vi "XYZMovingPartModifying_WangYunong.vi"() -> ()   [LabVIEW 2013]
uses:
  <vilib>/Math Plots/3D Math Plots/3D Bar/3D Bar XCtrl/3D Bar.xctl
  <vilib>/Math Plots/3D Math Plots/3D Bar/3D Bar Datatype/Public/Plot Helper (Matrix).vi
  <vilib>/Instr/_visa.llb/VISA Configure Serial Port (Instr).vi
  <vilib>/Math Plots/3D Math Plots/3D Bar/3D Bar Datatype/3D Bar Datatype.lvclass
panel:
  out "Zvel (mm/s)":dbl
  in  "stop":bool
  in  "Path":path
  out "Current ratio":dbl(graph)
  out "Surface Scanned":refnum<class "3D Plot Datatype.lvclass">[](xcontrol)
  in  "Z step / s":dbl format="%#_13g"
  out "Height / mm":dbl format="%#_13g"
  out "Present I Percent":dbl format="%#_13g"
  out "Present I / A":dbl format="%#_13g"
  in  "mm / step":dbl
  in  "ErrorTolerant %":dbl format="%#_13g"
  out "Reference A":dbl
  in  "VoltageGenerator":refnum<visa-resource-name>
  in  "ZMovingControl":refnum<visa-resource-name>
  out "Rod Pos?":cluster{dbl[], dbl[]}(graph)
  in  "X pole":refnum<visa-resource-name>
  in  "Y pole":refnum<visa-resource-name>
  in  "XYMov speed(mm/s)":dbl format="%#_13g"
  out "y resolution":dbl
  out "x resolution":dbl
  out "XY Graph":cluster{dbl[], dbl[]}(graph)
  in  "Y Center / mm":dbl format="%#_13g"
  in  "X Center / mm":dbl format="%#_13g"
  in  "Size input solution":enum16{"Dynamic Size", "Fixed Size"}(ring)=enum."Fixed Size"
  in  "Shape":enum16{"Self-defined", "Circle"}(ring)=enum."Circle"
  in  "Radius / mm":dbl format="%#_13g"
  in  "Precision":i32
  in  "Polygon Point":dbl[][](array[numeric])
  out "X":i32
  out "Y":i32
  in  "Y move Maximum / mm":dbl
  in  "X move Maximum / mm":dbl
  in  "Y step / mm":dbl
  in  "X step / mm":dbl
  in  "Initial YPos / mm":dbl
  in  "Initial XPos / mm":dbl
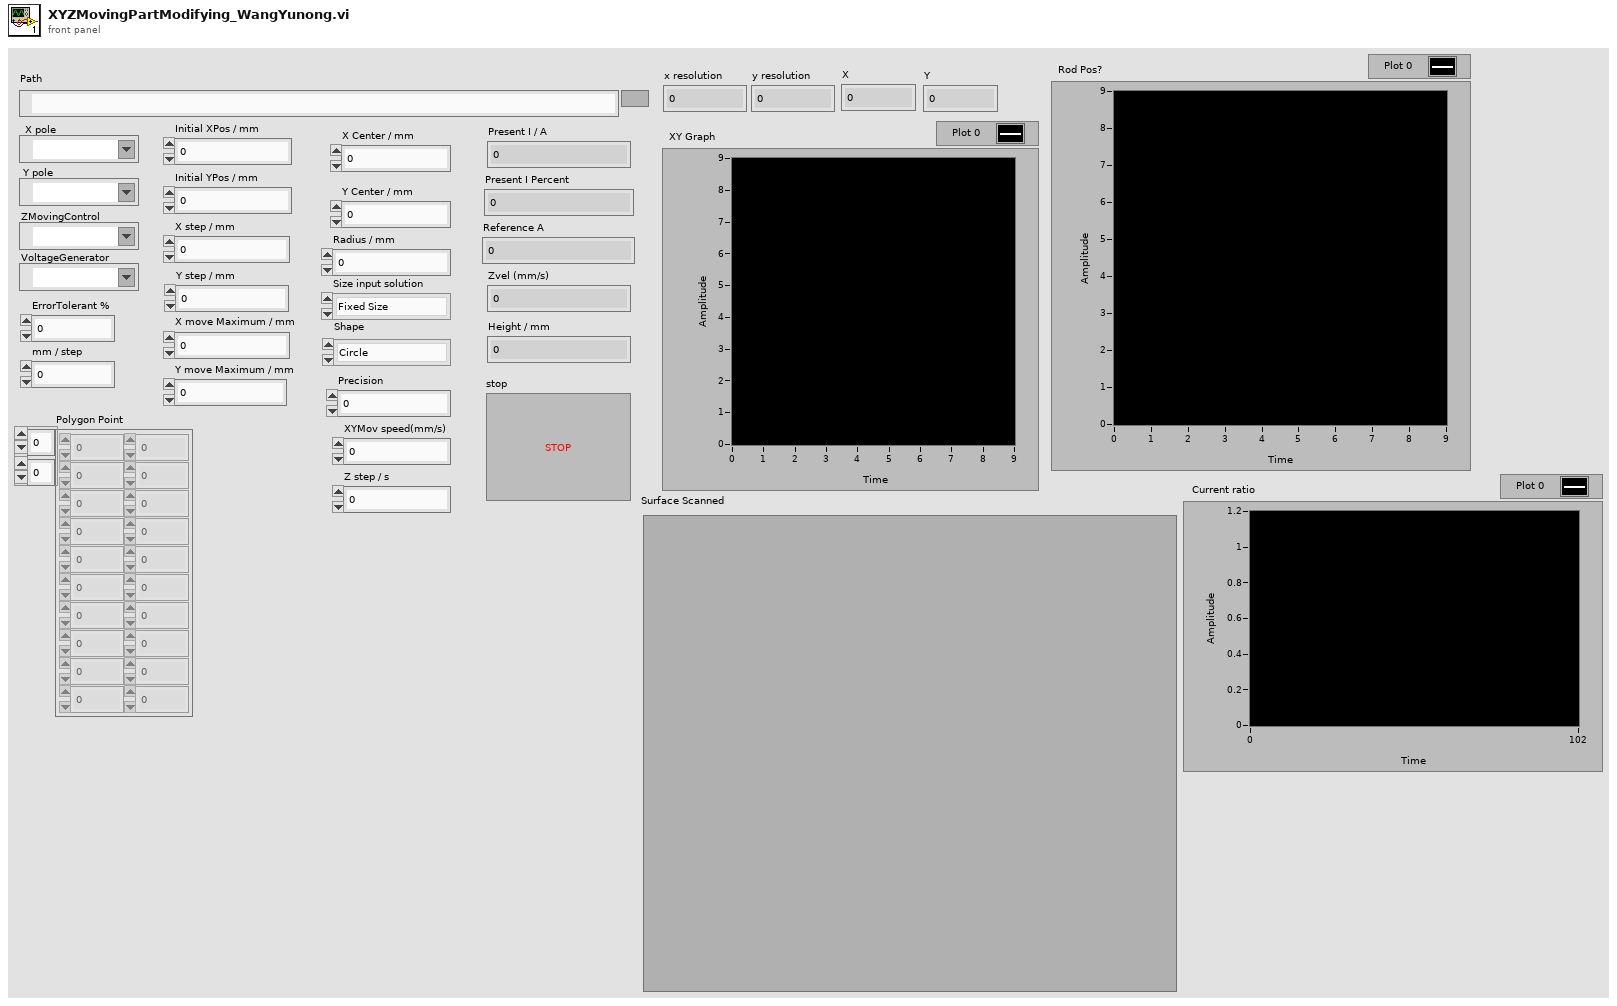
[diagram p1: front panel]
types:
  T1 = enum16{"open", "replace", "create", "open or create", "replace or create", "replace or create with confirmation"}
  T2 = typedef "NI_Matrix.lvlib/RealMatrix.ctl" = dbl[][]
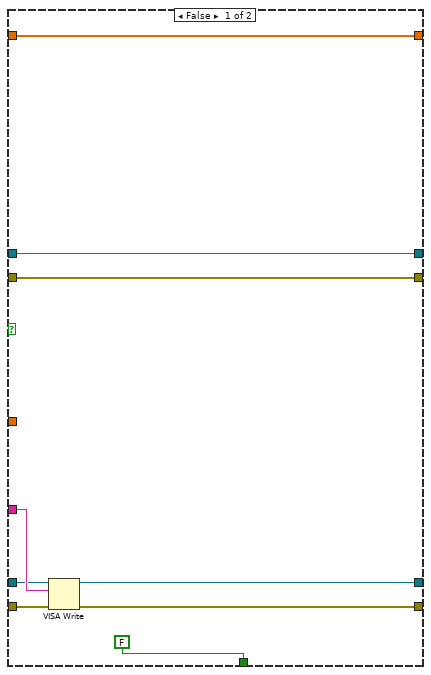
[diagram p3: hidden frame]
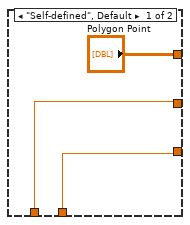
[diagram p4: hidden frame]
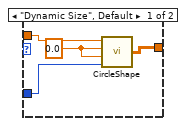
[diagram p5: hidden frame]
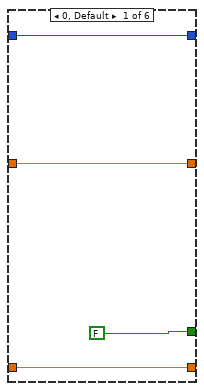
[diagram p6: hidden frame]
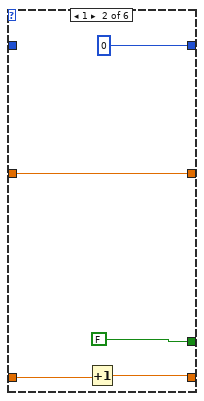
[diagram p7: hidden frame]
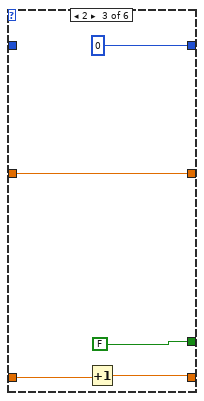
[diagram p8: hidden frame]
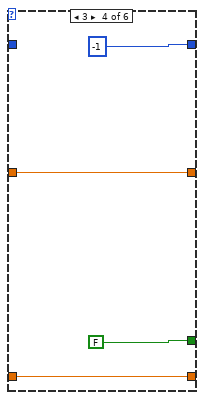
[diagram p9: hidden frame]
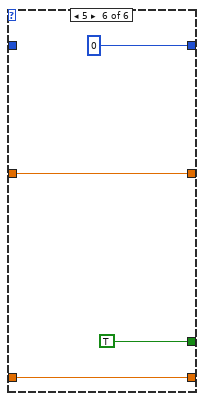
[diagram p10: hidden frame]
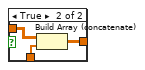
[diagram p11: hidden frame]
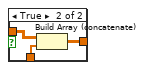
[diagram p12: hidden frame]
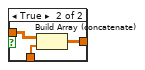
[diagram p13: hidden frame]
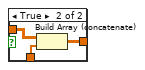
[diagram p14: hidden frame]
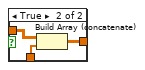
[diagram p15: hidden frame]
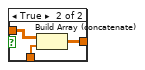
[diagram p16: hidden frame]
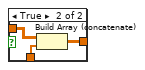
[diagram p17: hidden frame]
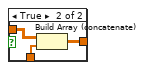
[diagram p18: hidden frame]
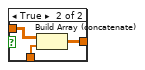
[diagram p19: hidden frame]
diagram:
  w59 = "ERR?\nMOV 1 0\n"
  w30 = dbl[] []
  w125 = 0 ("index")
  w94 = dbl[][] []
  w168 = 0
  w169 = 9.5
  w174 = 5.0
  # "sorted Y pos"
  # "sorted X pos"
  # "Control smallest step of 50nm"
  # "y length"
  # "x length"
  n1 = Greater?(x="Initial XPos / mm", y=w174) -> (0:w173:bool)
  n2 = Greater?(x="Initial YPos / mm", y=w174) -> (0:w172:bool)
  n3 = Or(x=w173, y=w172) -> (x .or. y?=w132:bool)
  n4 = case shown="True" w132 {
    tunnel: "Initial XPos / mm" -> [w176 _]
    tunnel: "Initial YPos / mm" -> [w175 _]
    tunnel: [w176 w177] -> w113
    tunnel: [w175 w177] -> w112
    frame False {
    }
    frame True {
      w177 = 5.0
    }
  }
  n5 = Greater Or Equal?(x=w112, y="Y move Maximum / mm") -> (x >= y?=w156:bool)
  n6 = Greater Or Equal?(x=w113, y="X move Maximum / mm") -> (x >= y?=w157:bool)
  n7 = Or(x=w157, y=w156) -> (x .or. y?=w131:bool)
  n8 = Less Or Equal?(x="Y step / mm", y=w168) -> (x <= y?=w165:bool)
  n9 = Greater Or Equal?(x="Y step / mm", y="Y move Maximum / mm") -> (x >= y?=w164:bool)
  n10 = Greater Or Equal?(x="X step / mm", y="X move Maximum / mm") -> (x >= y?=w166:bool)
  n11 = Less Or Equal?(x="X step / mm", y=w168) -> (x <= y?=w167:bool)
  n12 = Greater?(x="X move Maximum / mm", y=w169) -> (0:w155:bool)
  n13 = Greater?(x="Y move Maximum / mm", y=w169) -> (0:w154:bool)
  n14 = Compound Arithmetic op=OR(w167, w166, w165, w164) -> (w130:bool)
  n15 = case shown="True" w130 {
    tunnel: "X step / mm" -> [w179 _]
    tunnel: "Y step / mm" -> [w178 _]
    tunnel: [w179 w180] -> w153
    tunnel: [w178 w180] -> w152
    frame False {
    }
    frame True {
      w180 = 0.0
    }
  }
  n16 = case shown="True" w155 {
    tunnel: w169 -> [_ w182]
    tunnel: "X move Maximum / mm" -> [w181 _]
    tunnel: [w181 w182] -> w144
    frame False {
    }
    frame True {
    }
  }
  n17 = case shown="True" w154 {
    tunnel: w169 -> [_ w184]
    tunnel: "Y move Maximum / mm" -> [w183 _]
    tunnel: [w183 w184] -> w143
    frame False {
    }
    frame True {
    }
  }
  n18 = call "Intolerable Error 3"("Enable"=w130) -> ()  [unwired: 9 in, 2 out]
  n19 = call "Intolerable Error"("Enable"=w132) -> ()  [unwired: 9 in, 2 out]
  n20 = Subtract(x=w144, y=w113) -> (x-y=w138:dbl)
  n21 = Subtract(x=w143, y=w112) -> (x-y=w137:dbl)
  n22 = case shown="\"Circle\"" "Shape" {
    tunnel: ["Polygon Point" w200] -> w146
    tunnel: "Size input solution" -> [_ w199]
    tunnel: w138 -> [_ w195]
    tunnel: w137 -> [_ w194]
    tunnel: w112 -> [w185 w193]
    tunnel: w113 -> [w186 w192]
    tunnel: [w186 w191] -> w136
    tunnel: [w185 w190] -> w135
    tunnel: "X Center / mm" -> [_ w189]
    tunnel: "Y Center / mm" -> [_ w188]
    frame "Self-defined", Default {
    }
    frame "Circle" {
      w198 = 2.0
      n23 = Divide(x=w194, y=w198) -> (x/y=w196:dbl)
      n24 = Divide(x=w195, y=w198) -> (x/y=w197:dbl)
      n25 = case shown="\"Fixed Size\"" w199 {
        tunnel: "Radius / mm" -> [w205 w211]
        tunnel: "Precision" -> [w204 w210]
        tunnel: [w206 w209] -> w200
        tunnel: w189 -> [_ w208]
        tunnel: w188 -> [_ w207]
        frame "Dynamic Size", Default {
          w203 = 0.0 ("X initial")
          n26 = call "CircleShape.vi"("Precision"=w204, "Y initial"=w203, "X initial"=w203, "Radius"=w205) -> ("Output Point"=w206:dbl[][])
        }
        frame "Fixed Size" {
          n27 = call "CircleShape.vi"("Precision"=w210, "Y initial"=w207, "X initial"=w208, "Radius"=w211) -> ("Output Point"=w209:dbl[][])
        }
      }
      n28 = Add(x=w197, y=w192) -> (x+y=w191:dbl)
      n29 = Add(x=w196, y=w193) -> (x+y=w190:dbl)
    }
  }
  n30 = Index Array(array=w146, index (col)=1 ("disabled index (col)")) -> (element=w115:dbl[])  [unwired: 1 in]
  n31 = Index Array(array=w146, index (col)=0 ("disabled index (col)")) -> (element=w116:dbl[])  [unwired: 1 in]
  n32 = Array Size(array=w116) -> (size(s)=w118:i32)
  n33 = Array Size(array=w115) -> (size(s)=w117:i32)
  n34 = flat-sequence {
    tunnel: w153 -> [w225]
    tunnel: w152 -> [w222]
    tunnel: [w218] -> w54
    tunnel: [w217] -> w53
    frame #0 {
      w214 = 50
      w219 = 1000000.0
      n35 = Multiply(x=w219, y=w222) -> (x*y=w221:dbl)
      n36 = Multiply(x=w225, y=w219) -> (x*y=w224:dbl)
      n37 = Divide(x=w221, y=w214) -> (x/y=w220:dbl)
      n38 = Divide(x=w224, y=w214) -> (x/y=w223:dbl)
      n39 = Round To Nearest(number=w220) -> (nearest integer value=w215:dbl)
      n40 = Round To Nearest(number=w223) -> (nearest integer value=w216:dbl)
      n41 = Multiply(x=w215, y=w214) -> (x*y=w213:dbl)
      n42 = Multiply(x=w216, y=w214) -> (x*y=w212:dbl)
      n43 = Divide(x=w213, y=w219) -> (x/y=w217:dbl)
      n44 = Divide(x=w212, y=w219) -> (x/y=w218:dbl)
    }
  }
  n45 = call "Intolerable Error 4"("Enable"=w129) -> ()  [unwired: 9 in, 2 out]
  n46 = call "Intolerable Error 2"("Enable"=w131) -> ()  [unwired: 9 in, 2 out]
  n47 = call "Tolerable Error"("Enable"=w155) -> ()  [unwired: 9 in, 2 out]
  n48 = Sort 1D Array(array=w116) -> (sorted array=w123:dbl[])
  n49 = Sort 1D Array(array=w115) -> (sorted array=w124:dbl[])
  n50 = Decrement(x=w117) -> (x-1=w126:i32)
  n51 = Decrement(x=w118) -> (x-1=w127:i32)
  n52 = call "Tolerable Error 2"("Enable"=w154) -> ()  [unwired: 9 in, 2 out]
  n53 = Index Array(array=w123, index=w125) -> (element=w122:dbl)
  n54 = Index Array(array=w123, index=w127) -> (element=w121:dbl)
  n55 = Index Array(array=w124, index=w126) -> (element=w120:dbl)
  n56 = Index Array(array=w124, index=w125) -> (element=w119:dbl)
  n57 = flat-sequence {
    tunnel: w138 -> [w248]
    tunnel: w137 -> [w247]
    tunnel: w144 -> [w254]
    tunnel: w113 -> [w231]
    tunnel: w143 -> [w253]
    tunnel: w112 -> [w227]
    tunnel: [w252] -> w129
    tunnel: w54 -> [w230]
    tunnel: w53 -> [w226]
    tunnel: [w251] -> w3
    tunnel: [w229] -> w151
    tunnel: [w228] -> w150
    tunnel: [w226] -> w149
    tunnel: [w230] -> w148
    tunnel: [w246] -> w145
    tunnel: w136 -> [w245]
    tunnel: w135 -> [w244]
    tunnel: w144 -> [w243]
    tunnel: w143 -> [w242]
    tunnel: [w241] -> w140
    tunnel: [w240] -> w141
    tunnel: "Size input solution" -> [w239]
    tunnel: w122 -> [w238]
    tunnel: w121 -> [w237]
    tunnel: w120 -> [w236]
    tunnel: w119 -> [w235]
    tunnel: w116 -> [w234]
    tunnel: w115 -> [w233]
    tunnel: "Shape" -> [w232]
    tunnel: [w231] -> w103
    tunnel: [w230] -> w102
    tunnel: [w229] -> w101
    tunnel: [w228] -> w98
    tunnel: [w227] -> w97
    tunnel: [w226] -> w96
    frame #0 {
      n58 = case shown="\"Dynamic Size\", Default" w239 {
        tunnel: w234 -> [w277 w305]
        tunnel: w233 -> [w276 w304]
        tunnel: w237 -> [w283 w320]
        tunnel: w238 -> [w262 w318]
        tunnel: w236 -> [w282 w316]
        tunnel: w235 -> [w260 w313]
        tunnel: w248 -> [w281 _]
        tunnel: w247 -> [w278 _]
        tunnel: [w263 w306] -> w251
        tunnel: w254 -> [_ w319]
        tunnel: w231 -> [w271 w317]
        tunnel: w253 -> [_ w315]
        tunnel: w227 -> [w270 w314]
        tunnel: [FALSE w307] -> w252
        tunnel: w245 -> [w255 _]
        tunnel: w244 -> [w256 _]
        tunnel: w230 -> [w269 _]
        tunnel: w226 -> [w268 _]
        tunnel: [w266 w303] -> w241
        tunnel: [w267 w303] -> w240
        tunnel: w232 -> [w272 _]
        frame "Dynamic Size", Default {
          n59 = case shown="\"Self-defined\", Default" w272 {
            tunnel: w271 -> [_ w300]
            tunnel: w270 -> [_ w299]
            tunnel: w269 -> [_ w298]
            tunnel: w268 -> [_ w297]
            tunnel: [w289 w296] -> w267
            tunnel: [w289 w295] -> w266
            tunnel: w262 -> [w288 w294]
            tunnel: [w285 w293] -> w261
            tunnel: w260 -> [w287 w292]
            tunnel: [w284 w290] -> w259
            frame "Self-defined", Default {
              w286 = 0
              w289 = 0
              n60 = Multiply(x=w288, y=w286) -> (x*y=w285:dbl)
              n61 = Multiply(x=w286, y=w287) -> (x*y=w284:dbl)
            }
            frame "Circle" {
              w291 = 1.0
              n62 = Divide(x=w299, y=w297) -> (x/y=w301:dbl)
              n63 = Divide(x=w300, y=w298) -> (x/y=w302:dbl)
              n64 = Multiply(x=w294, y=w291) -> (x*y=w293:dbl)
              n65 = Multiply(x=w291, y=w292) -> (x*y=w290:dbl)
              n66 = Round Toward -Infinity(1:w302) -> (0:w296:dbl)
              n67 = Round Toward -Infinity(1:w301) -> (0:w295:dbl)
            }
          }
          n68 = Subtract(x=w282, y=w259) -> (x-y=w279:dbl)
          n69 = Subtract(x=w283, y=w261) -> (x-y=w280:dbl)
          n70 = Divide(x=w281, y=w280) -> (x/y=w258:dbl)
          n71 = Divide(x=w278, y=w279) -> (x/y=w257:dbl)
          n72 = Multiply(x=w258, y=w277) -> (x*y=w274:dbl[])
          n73 = Multiply(x=w257, y=w276) -> (x*y=w273:dbl[])
          n74 = Add(x=w274, y=w255) -> (x+y=w265:dbl[])
          n75 = Add(x=w273, y=w256) -> (x+y=w264:dbl[])
          n76 = Build Array(w265, w264) -> (w263:dbl[][])
        }
        frame "Fixed Size" {
          w303 = 0
          n77 = Greater?(x=w320, y=w319) -> (0:w311:bool)
          n78 = Less?(x=w318, y=w317) -> (x < y?=w312:bool)
          n79 = Greater?(x=w316, y=w315) -> (0:w310:bool)
          n80 = Less?(x=w313, y=w314) -> (x < y?=w309:bool)
          n81 = Compound Arithmetic op=OR(w312, w311, w310, w309) -> (w308:bool)
          n82 = case shown="True" w308 {
            tunnel: [FALSE TRUE] -> w307
            frame False {
            }
            frame True {
            }
          }
          n83 = Build Array(w305, w304) -> (w306:dbl[][])
        }
      }
      n84 = Divide(x=w243, y=w230) -> (x/y=w250:dbl)
      n85 = Divide(x=w242, y=w226) -> (x/y=w249:dbl)
      n86 = Round Toward -Infinity(1:w249) -> (0:w228:dbl)
      n87 = Round Toward -Infinity(1:w250) -> (0:w229:dbl)
      n88 = Get Date/Time In Seconds() -> (seconds since 1Jan1904=w246:timestamp)
    }
  }
  n89 = Compound Arithmetic op=OR(w132, w131, w130, w129, w60) -> (w128:bool)
  n90 = Stop(stop? (T)=w128) -> ()
  n91 = Divide(x=w97, y=w96) -> (x/y=w99:dbl)
  n92 = Divide(x=w103, y=w102) -> (x/y=w104:dbl)
  n93 = Round Toward -Infinity(1:w104) -> (0:w100:dbl)
  n94 = Round Toward -Infinity(1:w99) -> (0:w95:dbl)
  n95 = Subtract(x=w98, y=w95) -> (x-y=→"y resolution":dbl)
  n96 = Subtract(x=w101, y=w100) -> (x-y=→"x resolution":dbl)
  n97 = Transpose 2D Array(2D array=w3) -> (transposed array=w147:dbl[][])
  n98 = while {
    tunnel: w151 -> [w392]
    tunnel: w150 -> [w390]
    tunnel: w147 -> [w398]
    tunnel: w149 -> [w402]
    tunnel: w148 -> [w403]
    shift-right: [w383] -> _
    shift-left: 1 -> [w394]
    shift-right: [w382] -> _
    shift-left: w141 -> [w388]
    shift-right: [w381] -> _
    shift-left: w140 -> [w386]
    shift-right: [w380] -> w106
    shift-left: w94 -> [w397]
    tunnel: w141 -> [w378]
    shift-right: [w375] -> w105
    shift-left: w94 -> [w374]
    tunnel: w95 -> [w373]
    shift-right: [w368] -> w88
    shift-left: w94 -> [w370]
    shift-right: [w347] -> w87
    shift-left: w94 -> [w349]
    shift-right: [w344] -> w86
    shift-left: w94 -> [w346]
    shift-right: [w341] -> w85
    shift-left: w94 -> [w343]
    shift-right: [w338] -> w84
    shift-left: w94 -> [w340]
    shift-right: [w335] -> w82
    shift-left: w94 -> [w337]
    shift-right: [w332] -> w80
    shift-left: w94 -> [w334]
    shift-right: [w329] -> w79
    shift-left: w94 -> [w331]
    shift-right: [w326] -> w77
    shift-left: w94 -> [w328]
    shift-right: [w323] -> w74
    shift-left: w94 -> [w325]
    stop <- w385 stop-if-true
    w357 = 150.0
    n99 = Multiply(x=w403, y=w388) -> (x*y=w401:dbl)
    n100 = Multiply(x=w402, y=w386) -> (x*y=w400:dbl)
    n101 = Multiply(x=w357, y=3.0) -> (x*y=w367:dbl)
    n102 = Multiply(x=w357, y=2.0) -> (x*y=w372:dbl)
    n103 = Multiply(x=w357, y=4.0) -> (x*y=w363:dbl)
    n104 = Multiply(x=w357, y=5.0) -> (x*y=w356:dbl)
    n105 = Multiply(x=w357, y=8.0) -> (x*y=w353:dbl)
    n106 = Multiply(x=w357, y=6.0) -> (x*y=w355:dbl)
    n107 = Multiply(x=w357, y=10.0) -> (x*y=w351:dbl)
    n108 = Build Array(w401, w400) -> (w399:dbl[])
    n109 = Multiply(x=w357, y=7.0) -> (x*y=w354:dbl)
    n110 = Multiply(x=w357, y=9.0) -> (x*y=w352:dbl)
    n111 = Multiply(x=w357, y=11.0) -> (x*y=w350:dbl)
    n112 = flat-sequence {
      tunnel: w399 -> [w516]
      tunnel: w398 -> [w563]
      tunnel: w397 -> [w553]
      tunnel: [w566] -> w396
      tunnel: [w565] -> w395
      tunnel: w394 -> [w565]
      tunnel: [w485] -> w393
      tunnel: w392 -> [w486]
      tunnel: [w483] -> w391
      tunnel: w390 -> [w484]
      tunnel: [w564] -> w389
      tunnel: w388 -> [w564]
      tunnel: [w550] -> w387
      tunnel: w386 -> [w550]
      tunnel: [w561] -> w379
      tunnel: w378 -> [w561]
      tunnel: w357 -> [w554]
      tunnel: w372 -> [w555]
      tunnel: [w552] -> w376
      tunnel: w374 -> [w551]
      tunnel: w373 -> [w549]
      tunnel: w372 -> [w543]
      tunnel: w370 -> [w545]
      tunnel: [w544] -> w369
      tunnel: w367 -> [w515]
      tunnel: w363 -> [w513]
      tunnel: w356 -> [w512]
      tunnel: w355 -> [w511]
      tunnel: w354 -> [w510]
      tunnel: w353 -> [w509]
      tunnel: w352 -> [w508]
      tunnel: w351 -> [w507]
      tunnel: w350 -> [w505]
      tunnel: w349 -> [w504]
      tunnel: [w503] -> w348
      tunnel: w346 -> [w502]
      tunnel: [w501] -> w345
      tunnel: w343 -> [w500]
      tunnel: [w499] -> w342
      tunnel: w340 -> [w498]
      tunnel: [w497] -> w339
      tunnel: w337 -> [w496]
      tunnel: [w495] -> w336
      tunnel: w334 -> [w494]
      tunnel: [w493] -> w333
      tunnel: w331 -> [w492]
      tunnel: [w491] -> w330
      tunnel: w328 -> [w490]
      tunnel: [w489] -> w327
      tunnel: w325 -> [w488]
      tunnel: [w487] -> w324
      frame #0 {
        # "Max X step"
        # "Max Y step"
        # "Present y step Loc"
        # "Present x step Loc"
        # "Vx"
        n113 = Subtract(x=w550, y=w549) -> (x-y=w506:dbl)
        n114 = Less Or Equal?(x=w506, y=w507) -> (x <= y?=w520:bool)
        n115 = Less Or Equal?(x=w506, y=w509) -> (x <= y?=w524:bool)
        n116 = Less Or Equal?(x=w506, y=w508) -> (x <= y?=w522:bool)
        n117 = Less Or Equal?(x=w506, y=w511) -> (x <= y?=w528:bool)
        n118 = Less Or Equal?(x=w506, y=w510) -> (x <= y?=w526:bool)
        n119 = Less Or Equal?(x=w506, y=w505) -> (x <= y?=w518:bool)
        n120 = Less Or Equal?(x=w506, y=w512) -> (x <= y?=w530:bool)
        n121 = Less Or Equal?(x=w506, y=w515) -> (x <= y?=w547:bool)
        n122 = Less Or Equal?(x=w506, y=w513) -> (x <= y?=w532:bool)
        n123 = Less Or Equal?(x=w506, y=w555) -> (x <= y?=w557:bool)
        n124 = Greater?(x=w506, y=w511) -> (0:w525:bool)
        n125 = Greater?(x=w506, y=w509) -> (0:w521:bool)
        n126 = Greater?(x=w506, y=w510) -> (0:w523:bool)
        n127 = Greater?(x=w506, y=w508) -> (0:w519:bool)
        n128 = Greater?(x=w506, y=w513) -> (0:w529:bool)
        n129 = Greater?(x=w506, y=w515) -> (0:w531:bool)
        n130 = Greater?(x=w506, y=w512) -> (0:w527:bool)
        n131 = Greater?(x=w506, y=w507) -> (0:w517:bool)
        n132 = Greater?(x=w506, y=w543) -> (0:w546:bool)
        n133 = Greater?(x=w506, y=w505) -> (0:w514:bool)
        n134 = Less Or Equal?(x=w506, y=w554) -> (x <= y?=w559:bool)
        n135 = Greater?(x=w506, y=w554) -> (0:w556:bool)
        n136 = call "WhetherInnerOrOn.vi"("Error permitted"=0.0001, "JudgePoint"=w516, "InputPolygon"=w563) -> ("Point on or inside?"=w533:bool)
        n137 = Compound Arithmetic op=AND(w533, w547, w546) -> (w548:bool)
        n138 = Compound Arithmetic op=AND(w533, w530, w529) -> (w541:bool)
        n139 = And(x=w533, y=w559) -> (x .and. y?=w560:bool)
        n140 = Compound Arithmetic op=AND(w533, w532, w531) -> (w542:bool)
        n141 = Compound Arithmetic op=AND(w533, w528, w527) -> (w540:bool)
        n142 = Compound Arithmetic op=AND(w533, w526, w525) -> (w539:bool)
        n143 = Compound Arithmetic op=AND(w533, w524, w523) -> (w538:bool)
        n144 = Compound Arithmetic op=AND(w533, w522, w521) -> (w537:bool)
        n145 = Compound Arithmetic op=AND(w533, w557, w556) -> (w558:bool)
        n146 = Compound Arithmetic op=AND(w533, w520, w519) -> (w536:bool)
        n147 = Compound Arithmetic op=AND(w533, w518, w517) -> (w535:bool)
        n148 = Compound Arithmetic op=AND(w533, w514) -> (w534:bool)
        n149 = Decrement(x=w486) -> (x-1=w485:dbl)
        n150 = Decrement(x=w484) -> (x-1=w483:dbl)
        n151 = case shown="True" w560 {
          tunnel: w553 -> [w611 w614]
          tunnel: w516 -> [_ w613]
          tunnel: [w611 w612] -> w566
          frame False {
          }
          frame True {
            n152 = Build Array (concatenate)(w614, w613) -> (w612:dbl[][])
          }
        }
        n153 = case shown="True" w558 {
          tunnel: w516 -> [_ w610]
          tunnel: w551 -> [w607 w609]
          tunnel: [w607 w608] -> w552
          frame False {
          }
          frame True {
            n154 = Build Array (concatenate)(w609, w610) -> (w608:dbl[][])
          }
        }
        n155 = case shown="True" w548 {
          tunnel: w516 -> [_ w606]
          tunnel: w545 -> [w603 w605]
          tunnel: [w603 w604] -> w544
          frame False {
          }
          frame True {
            n156 = Build Array (concatenate)(w605, w606) -> (w604:dbl[][])
          }
        }
        n157 = case shown="False" w541 {
          tunnel: w516 -> [_ w570]
          tunnel: [w567 w569] -> w501
          tunnel: w502 -> [w567 w568]
          frame False {
          }
          frame True {
            n158 = Build Array (concatenate)(w568, w570) -> (w569:dbl[][])
          }
        }
        n159 = case shown="False" w542 {
          tunnel: w516 -> [_ w602]
          tunnel: [w599 w601] -> w503
          tunnel: w504 -> [w599 w600]
          frame False {
          }
          frame True {
            n160 = Build Array (concatenate)(w600, w602) -> (w601:dbl[][])
          }
        }
        n161 = case shown="False" w539 {
          tunnel: w516 -> [_ w594]
          tunnel: [w591 w593] -> w497
          tunnel: w498 -> [w591 w592]
          frame False {
          }
          frame True {
            n162 = Build Array (concatenate)(w592, w594) -> (w593:dbl[][])
          }
        }
        n163 = case shown="False" w540 {
          tunnel: w516 -> [_ w598]
          tunnel: [w595 w597] -> w499
          tunnel: w500 -> [w595 w596]
          frame False {
          }
          frame True {
            n164 = Build Array (concatenate)(w596, w598) -> (w597:dbl[][])
          }
        }
        n165 = case shown="False" w537 {
          tunnel: w516 -> [_ w586]
          tunnel: [w583 w585] -> w493
          tunnel: w494 -> [w583 w584]
          frame False {
          }
          frame True {
            n166 = Build Array (concatenate)(w584, w586) -> (w585:dbl[][])
          }
        }
        n167 = case shown="False" w538 {
          tunnel: w516 -> [_ w590]
          tunnel: [w587 w589] -> w495
          tunnel: w496 -> [w587 w588]
          frame False {
          }
          frame True {
            n168 = Build Array (concatenate)(w588, w590) -> (w589:dbl[][])
          }
        }
        n169 = case shown="False" w536 {
          tunnel: w516 -> [_ w582]
          tunnel: [w579 w581] -> w491
          tunnel: w492 -> [w579 w580]
          frame False {
          }
          frame True {
            n170 = Build Array (concatenate)(w580, w582) -> (w581:dbl[][])
          }
        }
        n171 = case shown="False" w535 {
          tunnel: w516 -> [_ w578]
          tunnel: [w575 w577] -> w489
          tunnel: w490 -> [w575 w576]
          frame False {
          }
          frame True {
            n172 = Build Array (concatenate)(w576, w578) -> (w577:dbl[][])
          }
        }
        n173 = case shown="False" w534 {
          tunnel: w516 -> [_ w574]
          tunnel: [w571 w573] -> w487
          tunnel: w488 -> [w571 w572]
          frame False {
          }
          frame True {
            n174 = Build Array (concatenate)(w572, w574) -> (w573:dbl[][])
          }
        }
      }
    }
    n175 = flat-sequence {
      tunnel: w396 -> [w419]
      tunnel: w395 -> [w426]
      tunnel: w393 -> [w456]
      tunnel: w391 -> [w454]
      tunnel: w389 -> [w425]
      tunnel: w387 -> [w424]
      tunnel: [w423] -> w385
      tunnel: [w422] -> w384
      tunnel: [w421] -> w383
      tunnel: [w420] -> w381
      tunnel: [w419] -> w380
      tunnel: w379 -> [w418]
      tunnel: w376 -> [w414]
      tunnel: [w414] -> w375
      tunnel: w369 -> [w413]
      tunnel: [w413] -> w368
      tunnel: [w412] -> w347
      tunnel: w348 -> [w412]
      tunnel: w345 -> [w411]
      tunnel: [w411] -> w344
      tunnel: w342 -> [w410]
      tunnel: [w410] -> w341
      tunnel: w339 -> [w409]
      tunnel: [w409] -> w338
      tunnel: w336 -> [w408]
      tunnel: [w408] -> w335
      tunnel: w333 -> [w407]
      tunnel: [w407] -> w332
      tunnel: w330 -> [w406]
      tunnel: [w406] -> w329
      tunnel: w327 -> [w405]
      tunnel: [w405] -> w326
      tunnel: w324 -> [w404]
      tunnel: [w404] -> w323
      frame #0 {
        w416 = 0.0
        # "Case5"
        # "Case4"
        # "Case3"
        # "Case2"
        # "Case1"
        n176 = Equal?(x=w425, y=w456) -> (x = y?=w446:bool)
        n177 = Equal?(x=w425, y=w418) -> (x = y?=w447:bool)
        n178 = Equal?(x=w424, y=w454) -> (x = y?=w448:bool)
        n179 = Less?(x=w424, y=w454) -> (x < y?=w452:bool)
        n180 = Equal?(x=w426, y=1.0) -> (x = y?=w455:bool)
        n181 = Equal?(x=w426, y=w416) -> (x = y?=w451:bool)
        n182 = Equal?(x=w426, y=-1.0) -> (x = y?=w453:bool)
        n183 = Not Equal?(x=w426, y=w416) -> (x != y?=w449:bool)
        n184 = Or(x=w447, y=w446) -> (x .or. y?=w450:bool)
        n185 = Compound Arithmetic op=AND(w455, w446, w452) -> (w445:bool)
        n186 = Compound Arithmetic op=AND(w451, w446) -> (w443:bool)
        n187 = Compound Arithmetic op=AND(w453, w447, w452) -> (w444:bool)
        n188 = Compound Arithmetic op=AND(w451, w447) -> (w442:bool)
        n189 = Compound Arithmetic op=AND(w450, w448, w449) -> (w441:bool)
        n190 = Boolean To (0,1)(Boolean=w443) -> (0, 1=w436:i16)
        n191 = Boolean To (0,1)(Boolean=w442) -> (0, 1=w434:i16)
        n192 = Boolean To (0,1)(Boolean=w444) -> (0, 1=w438:i16)
        n193 = Boolean To (0,1)(Boolean=w445) -> (0, 1=w439:i16)
        n194 = Boolean To (0,1)(Boolean=w441) -> (0, 1=w432:i16)
        n195 = Multiply(x=w438, y=i16 2) -> (x*y=w430:i16)
        n196 = Multiply(x=w436, y=i16 3) -> (x*y=w429:i16)
        n197 = Multiply(x=w434, y=i16 4) -> (x*y=w428:i16)
        n198 = Multiply(x=w432, y=i16 5) -> (x*y=w427:i16)
        n199 = Compound Arithmetic op=ADD(w439, w430, w429, w428, w427) -> (w440:i16)
        n200 = case shown="4" w440 {
          tunnel: w426 -> [w460 _ _ _ _ _]
          tunnel: w425 -> [w459 w462 w467 w473 w477 w482]
          tunnel: w424 -> [w458 w464 w469 w472 w476 w481]
          tunnel: [w460 0 0 -1 1 0] -> w421
          tunnel: [w459 w462 w467 w473 w477 w482] -> w422
          tunnel: [w458 w463 w468 w472 w476 w481] -> w420
          tunnel: [FALSE FALSE FALSE FALSE FALSE TRUE] -> w423
          frame 0, Default {
          }
          frame 1 {
            n201 = Increment(x=w464) -> (x+1=w463:dbl)
          }
          frame 2 {
            n202 = Increment(x=w469) -> (x+1=w468:dbl)
          }
          frame 3 {
          }
          frame 4 {
          }
          frame 5 {
          }
        }
        "X" <- w425
        "Y" <- w424
      }
    }
    n203 = Add(x=w383, y=w384) -> (x+y=w382:dbl)
  }
  n204 = Insert Into Array(array=w106, new element=w105) -> (w93:dbl[][])  [unwired: 2 in]
  n205 = Insert Into Array(array=w93, new element=w88) -> (w92:dbl[][])  [unwired: 2 in]
  n206 = Insert Into Array(array=w92, new element=w87) -> (w91:dbl[][])  [unwired: 2 in]
  n207 = Insert Into Array(array=w91, new element=w86) -> (w90:dbl[][])  [unwired: 2 in]
  n208 = Insert Into Array(array=w90, new element=w85) -> (w89:dbl[][])  [unwired: 2 in]
  n209 = Insert Into Array(array=w89, new element=w84) -> (w83:dbl[][])  [unwired: 2 in]
  n210 = Insert Into Array(array=w83, new element=w82) -> (w81:dbl[][])  [unwired: 2 in]
  n211 = Insert Into Array(array=w81, new element=w80) -> (w78:dbl[][])  [unwired: 2 in]
  n212 = Insert Into Array(array=w78, new element=w79) -> (w76:dbl[][])  [unwired: 2 in]
  n213 = Insert Into Array(array=w76, new element=w77) -> (w75:dbl[][])  [unwired: 2 in]
  n214 = Insert Into Array(array=w75, new element=w74) -> (w73:dbl[][])  [unwired: 2 in]
  n215 = flat-sequence {
    tunnel: [w618] -> w52
    tunnel: w73 -> [w618]
    tunnel: w145 -> [w617]
    tunnel: [w616] -> _
    tunnel: [w615] -> w43
    frame #0 {
      n216 = Get Date/Time In Seconds() -> (seconds since 1Jan1904=w615:timestamp)
      n217 = Subtract(x=w615, y=w617) -> (x-y=w616:dbl)
    }
  }
  n218 = Index Array(array=w52, index (col)=0 ("disabled index (col)")) -> (element=w109:dbl[])  [unwired: 1 in]
  n219 = Index Array(array=w52, index (col)=1 ("disabled index (col)")) -> (element=w110:dbl[])  [unwired: 1 in]
  n220 = Bundle(w109, w110) -> (→"XY Graph":cluster{dbl[], dbl[]})  [unwired: 1 in]
  n221 = flat-sequence {
    tunnel: [w686] -> w72
    tunnel: w52 -> [w686]
    tunnel: [w679] -> w71
    tunnel: [w678] -> w70
    tunnel: [w683] -> w69
    tunnel: [w682] -> w68
    tunnel: [w672] -> w60
    tunnel: ["XYMov speed(mm/s)"] -> w62
    tunnel: [w646] -> w42
    tunnel: [w645] -> w41
    tunnel: [w633] -> w40
    tunnel: [w632] -> w39
    tunnel: ["mm / step"] -> w2
    frame #0 {
      w687 = "ERR?\nSVO 1 1\nMOV 1 0\n"
      n222 = Multiply(x="Z step / s", y="mm / step") -> (x*y=w620:dbl)
      "Zvel (mm/s)" <- w620
      n223 = call-poly "VISA Configure Serial Port"("VISA resource name"="ZMovingControl", "baud rate (9600)"=u32 115200) -> ("VISA resource name out"=w626:refnum<visa-resource-name>, "error out"=w625:errorcluster)  [unwired: 12 in]
      n224 = Number To Fractional String(number=w620) -> (F-format string=w655:string)  [unwired: 3 in]
      n225 = call-poly "VISA Configure Serial Port"("VISA resource name"="VoltageGenerator", "baud rate (9600)"=57600) -> ("VISA resource name out"=w642:refnum<visa-resource-name>, "error out"=w641:errorcluster)  [unwired: 12 in]
      n226 = Concatenate Strings("VEL 1 ", w655, "\n" ("string")) -> (w652:string)
      n227 = call-poly "VISA Configure Serial Port"("VISA resource name"="Y pole", "baud rate (9600)"=u32 115200) -> ("VISA resource name out"=w628:refnum<visa-resource-name>, "error out"=w627:errorcluster)  [unwired: 12 in]
      n228 = VISA Write(VISA resource name=w626, write buffer=w652, error in (no error)=w625) -> (VISA resource name out=w657:refnum<visa-resource-name>, error out=w656:errorcluster)  [unwired: 1 out]
      n229 = VISA Write(VISA resource name=w642, write buffer=":SYST:PRES\n", error in (no error)=w641) -> (VISA resource name out=w640:refnum<visa-resource-name>, error out=w639:errorcluster)  [unwired: 1 out]
      n230 = VISA Write(VISA resource name=w657, write buffer="ERR?\nPOS?\n", error in (no error)=w656) -> (VISA resource name out=w662:refnum<visa-resource-name>, error out=w661:errorcluster)  [unwired: 1 out]
      n231 = call-poly "VISA Configure Serial Port"("VISA resource name"="X pole", "baud rate (9600)"=u32 115200) -> ("VISA resource name out"=w630:refnum<visa-resource-name>, "error out"=w629:errorcluster)  [unwired: 12 in]
      n232 = local write "Zvel (mm/s)"(w620) -> ()
      n233 = VISA Write(VISA resource name=w640, write buffer=":SENS:FUNC 'CURR'\n:SENS:CURR:RANG:AUTO 1\n:SENS:CURR:NPLC 0.1\n:OUTP 1\n:SOUR:VOLT 0.2\n:SYST:ZCH OFF\n", error in (no error)=w639) -> (VISA resource name out=w667:refnum<visa-resource-name>, error out=w666:errorcluster)  [unwired: 1 out]
      n234 = VISA Read(VISA resource name=w662, byte count=128, error in (no error)=w661) -> (VISA resource name out=w659:refnum<visa-resource-name>, read buffer=w651:string, error out=w658:errorcluster)  [unwired: 1 out]
      n235 = Fract/Exp String To Number(string=w651, offset=8) -> (number=w649:dbl)  [unwired: 2 in, 1 out]
      n236 = Number To Fractional String(number="XYMov speed(mm/s)", precision (6)=i16 12) -> (F-format string=w676:string)  [unwired: 2 in]
      n237 = Divide(x=w649, y=w620) -> (x/y=w623:dbl)
      n238 = VISA Write(VISA resource name=w659, write buffer="SVO 1 1\nMOV 1 0\n", error in (no error)=w658) -> (VISA resource name out=w647:refnum<visa-resource-name>, error out=w644:errorcluster)  [unwired: 1 out]
      n239 = VISA Write(VISA resource name=w667, write buffer=":DATA:FRES?\n", error in (no error)=w666) -> (VISA resource name out=w635:refnum<visa-resource-name>, error out=w634:errorcluster)  [unwired: 1 out]
      n240 = Equal To 0?(x="XYMov speed(mm/s)") -> (x = 0?=w672:bool)
      n241 = Multiply(x=w623, y=1000) -> (x*y=w624:dbl)
      n242 = VISA Write(VISA resource name=w628, write buffer=w687, error in (no error)=w627) -> (VISA resource name out=w685:refnum<visa-resource-name>, error out=w684:errorcluster)  [unwired: 1 out]
      n243 = VISA Write(VISA resource name=w630, write buffer=w687, error in (no error)=w629) -> (VISA resource name out=w681:refnum<visa-resource-name>, error out=w680:errorcluster)  [unwired: 1 out]
      n244 = Add(x=w624, y=1000) -> (x+y=w643:dbl)
      n245 = Concatenate Strings("VEL 1 ", w676, "\n") -> (w673:string)
      n246 = flat-sequence {
        tunnel: w647 -> [w694]
        tunnel: [w694] -> w646
        tunnel: [w693] -> w645
        tunnel: w644 -> [w693]
        tunnel: w643 -> [w692]
        frame #0 {
          n247 = Wait (ms)(milliseconds to wait=w692) -> ()  [unwired: 1 out]
        }
      }
      n248 = VISA Read(VISA resource name=w635, byte count=u32 128, error in (no error)=w634) -> (VISA resource name out=w633:refnum<visa-resource-name>, error out=w632:errorcluster)  [unwired: 2 out]
      n249 = VISA Write(VISA resource name=w685, write buffer=w673, error in (no error)=w684) -> (VISA resource name out=w683:refnum<visa-resource-name>, error out=w682:errorcluster)  [unwired: 1 out]
      n250 = VISA Write(VISA resource name=w681, write buffer=w673, error in (no error)=w680) -> (VISA resource name out=w679:refnum<visa-resource-name>, error out=w678:errorcluster)  [unwired: 1 out]
    }
  }
  n251 = flat-sequence {
    tunnel: [w743] -> w67
    tunnel: w72 -> [w743]
    tunnel: [w750] -> w66
    tunnel: w71 -> [w751]
    tunnel: w70 -> [w749]
    tunnel: [w748] -> w65
    tunnel: w69 -> [w747]
    tunnel: [w746] -> w64
    tunnel: [w744] -> w63
    tunnel: w68 -> [w745]
    tunnel: w62 -> [w723]
    tunnel: [w723] -> w61
    tunnel: w42 -> [w709]
    tunnel: w41 -> [w708]
    tunnel: w40 -> [w722]
    tunnel: w39 -> [w721]
    tunnel: [w717] -> w35
    tunnel: [w716] -> w34
    tunnel: [w704] -> w38
    tunnel: [w710] -> w37
    tunnel: [w701] -> w36
    tunnel: [w709] -> w33
    tunnel: [w708] -> w32
    tunnel: [w696] -> w31
    tunnel: [w702] -> w4
    tunnel: w2 -> [w696]
    tunnel: [w695] -> w1
    frame #0 {
      w695 = 0.05
      w706 = 1
      # "Z scan limit / mm"
      n252 = Index Array(array=w743, index (row)=0) -> (element=w729:dbl[])  [unwired: 1 in]
      n253 = Index Array(array=w729, index=1) -> (element=w728:dbl)
      n254 = Index Array(array=w729, index=0) -> (element=w727:dbl)
      n255 = Max & Min(x=w728, y=w727) -> (max(x,y)=w724:dbl)  [unwired: 1 out]
      n256 = Divide(x="ErrorTolerant %", y=100.0) -> (x/y=w705:dbl)
      n257 = Divide(x=w724, y=w723) -> (x/y=w700:dbl)
      n258 = VISA Write(VISA resource name=w722, write buffer=":DATA:FRES?\n", error in (no error)=w721) -> (VISA resource name out=w719:refnum<visa-resource-name>, error out=w718:errorcluster)  [unwired: 1 out]
      n259 = Number To Fractional String(number=w728, precision (6)=i16 10) -> (F-format string=w735:string)  [unwired: 2 in]
      n260 = Concatenate Strings("MOV 1 ", w735, "\n" ("string")) -> (w732:string)
      n261 = Number To Fractional String(number=w727, precision (6)=i16 10) -> (F-format string=w740:string)  [unwired: 2 in]
      n262 = Concatenate Strings("MOV 1 ", w740, "\n" ("string")) -> (w737:string)
      n263 = Add(x=w706, y=w705) -> (x+y=w703:dbl)
      n264 = Subtract(x=w706, y=w705) -> (x-y=w711:dbl)
      n265 = VISA Read(VISA resource name=w719, byte count=u32 128, error in (no error)=w718) -> (VISA resource name out=w717:refnum<visa-resource-name>, read buffer=w715:string, error out=w716:errorcluster)  [unwired: 1 out]
      n266 = VISA Write(VISA resource name=w747, write buffer=w732, error in (no error)=w745) -> (VISA resource name out=w746:refnum<visa-resource-name>, error out=w744:errorcluster)  [unwired: 1 out]
      n267 = Multiply(x=w700, y=1000) -> (x*y=w698:dbl)
      n268 = VISA Write(VISA resource name=w751, write buffer=w737, error in (no error)=w749) -> (VISA resource name out=w750:refnum<visa-resource-name>, error out=w748:errorcluster)  [unwired: 1 out]
      n269 = Fract/Exp String To Number(string=w715, offset=1) -> (number=w704:dbl)  [unwired: 2 in, 1 out]
      "Reference A" <- w704
      n270 = Add(x=w698, y=u32 2000 ("milliseconds to wait")) -> (x+y=w726:dbl)
      n271 = Multiply(x=w704, y=w711) -> (x*y=w710:dbl)
      n272 = Wait (ms)(milliseconds to wait=w726) -> ()  [unwired: 1 out]
      n273 = Multiply(x=w704, y=w703) -> (x*y=w702:dbl)
      n274 = Divide(x=w695, y=w696) -> (x/y=w697:dbl)
      n275 = Round Toward -Infinity(1:w697) -> (0:w701:dbl)
    }
  }
  n276 = call <vilib>:"Check if File or Folder Exists.vi"("path"="Path") -> ("file or folder exists?"=w22:bool)  [unwired: 8 in, 2 out]
  n277 = case shown="True" w22 {
    tunnel: "Path" -> [w752 w754]
    tunnel: [w752 w753] -> w19
    frame False {
    }
    frame True {
      n278 = Delete(path (use dialog)=w754) -> (deleted path=w753:path)  [unwired: 4 in, 2 out]
    }
  }
  n279 = Open/Create/Replace File(file path (use dialog)=w19, operation (0:open)=T1."create") -> (refnum out=w18:refnum<file>, error out=w17:errorcluster)  [unwired: 4 in, 1 out]
  n280 = while {
    tunnel: w67 -> [w866]
    tunnel: w66 -> [w870]
    tunnel: w65 -> [w869]
    tunnel: w64 -> [w868]
    tunnel: w63 -> [w867]
    shift-right: [w837] -> w28
    shift-left: w30 -> [w855]
    tunnel: w61 -> [w852]
    tunnel: [w764] -> w50
    tunnel: [w763] -> w48
    tunnel: [w848] -> w46
    tunnel: [w847] -> w44
    shift-right: [w835] -> w27
    shift-left: w30 -> [w836]
    tunnel: w54 -> [w833]
    tunnel: w53 -> [w834]
    tunnel: w38 -> [w801]
    tunnel: w37 -> [w830]
    tunnel: w36 -> [w829]
    tunnel: w35 -> [w821]
    tunnel: w34 -> [w818]
    tunnel: w33 -> [w815]
    tunnel: w32 -> [w812]
    tunnel: w31 -> [w809]
    shift-right: [w795] -> w25
    shift-left: w30 -> [w794]
    tunnel: w18 -> [w779]
    tunnel: w17 -> [w778]
    tunnel: [w777] -> w16
    tunnel: [w776] -> w15
    tunnel: [w775] -> w9
    tunnel: [w774] -> w8
    tunnel: [w773] -> w14
    tunnel: [w772] -> w13
    tunnel: w4 -> [w771]
    tunnel: w1 -> [w758]
    i -> [w865]
    stop <- w767 stop-if-true
    # "x"
    # "Scanner"
    # "Spare for Z mov part"
    n281 = Index Array(array=w866, index (col)=0 ("disabled index (col)")) -> (element=w871:dbl[])  [unwired: 1 in]
    n282 = Index Array(array=w866, index (row)=w865) -> (element=w858:dbl[])  [unwired: 1 in]
    n283 = Index Array(array=w858, index=0) -> (element=w854:dbl)
    n284 = Index Array(array=w858, index=1) -> (element=w853:dbl)
    n285 = Array Size(array=w871) -> (size(s)=w831:i32)
    n286 = flat-sequence {
      tunnel: w870 -> [w1102]
      tunnel: w869 -> [w1101]
      tunnel: w868 -> [w1090]
      tunnel: w867 -> [w1089]
      tunnel: [w1074] -> w864
      tunnel: [w1073] -> w863
      tunnel: [w1070] -> w860
      tunnel: [w1069] -> w861
      tunnel: w854 -> [w1095]
      tunnel: w853 -> [w1087]
      tunnel: w830 -> [w1085]
      tunnel: w829 -> [w1086]
      tunnel: [w1086] -> w827
      tunnel: [w1085] -> w824
      tunnel: [w1084] -> w822
      tunnel: w821 -> [w1084]
      tunnel: [w1083] -> w819
      tunnel: w818 -> [w1083]
      tunnel: [w1082] -> w816
      tunnel: w815 -> [w1082]
      tunnel: [w1081] -> w813
      tunnel: w812 -> [w1081]
      tunnel: [w1080] -> w810
      tunnel: w809 -> [w1080]
      tunnel: [w1079] -> w802
      tunnel: w801 -> [w1079]
      tunnel: [w1078] -> w796
      tunnel: w794 -> [w1078]
      tunnel: w771 -> [w1077]
      tunnel: [w1077] -> w769
      tunnel: w758 -> [w1068]
      tunnel: [w1068] -> w757
      frame #0 {
        n287 = Number To Fractional String(number=w1095, precision (6)=i16 12) -> (F-format string=w1098:string)  [unwired: 2 in]
        n288 = Number To Fractional String(number=w1087, precision (6)=i16 12) -> (F-format string=w1093:string)  [unwired: 2 in]
        n289 = Concatenate Strings("MOV 1 ", w1098, "\n") -> (w1100:string)
        n290 = Concatenate Strings("MOV 1 ", w1093, "\n" ("string")) -> (w1088:string)
        n291 = VISA Write(VISA resource name=w1102, write buffer=w1100, error in (no error)=w1101) -> (VISA resource name out=w1076:refnum<visa-resource-name>, error out=w1075:errorcluster)  [unwired: 1 out]
        n292 = VISA Write(VISA resource name=w1090, write buffer=w1088, error in (no error)=w1089) -> (VISA resource name out=w1072:refnum<visa-resource-name>, error out=w1071:errorcluster)  [unwired: 1 out]
        n293 = VISA Flush I/O Buffer(VISA resource name=w1076, error in (no error)=w1075) -> (VISA resource name out=w1074:refnum<visa-resource-name>, error out=w1073:errorcluster)  [unwired: 1 in]
        n294 = VISA Flush I/O Buffer(VISA resource name=w1072, error in (no error)=w1071) -> (VISA resource name out=w1070:refnum<visa-resource-name>, error out=w1069:errorcluster)  [unwired: 1 in]
      }
    }
    n295 = Equal?(x=w865, y=w831) -> (x = y?=w766:bool)
    n296 = Max & Min(x=w833, y=w834) -> (max(x,y)=w832:dbl)  [unwired: 1 out]
    n297 = Divide(x=w832, y=w852) -> (x/y=w762:dbl)
    n298 = Multiply(x=w762, y=1000) -> (x*y=w760:dbl)
    n299 = Add(x=w760, y=100) -> (x+y=w840:dbl)
    n300 = flat-sequence {
      tunnel: w864 -> [w1036]
      tunnel: w863 -> [w1035]
      tunnel: w861 -> [w1033]
      tunnel: w860 -> [w1034]
      tunnel: [w1036] -> w844
      tunnel: [w1035] -> w843
      tunnel: [w1034] -> w842
      tunnel: [w1033] -> w841
      tunnel: w840 -> [w1032]
      tunnel: [w1031] -> w828
      tunnel: w827 -> [w1031]
      tunnel: [w1030] -> w825
      tunnel: w824 -> [w1030]
      tunnel: [w1029] -> w823
      tunnel: w822 -> [w1029]
      tunnel: [w1028] -> w820
      tunnel: w819 -> [w1028]
      tunnel: [w1027] -> w817
      tunnel: w816 -> [w1027]
      tunnel: [w1026] -> w814
      tunnel: w813 -> [w1026]
      tunnel: [w1025] -> w811
      tunnel: w810 -> [w1025]
      tunnel: w802 -> [w1024]
      tunnel: [w1024] -> w799
      tunnel: [w1023] -> w797
      tunnel: w796 -> [w1023]
      tunnel: [w1022] -> w770
      tunnel: w769 -> [w1022]
      tunnel: w757 -> [w1021]
      tunnel: [w1021] -> w755
      tunnel: [w1064] -> w846
      tunnel: [w1065] -> w849
      tunnel: [w1066] -> w850
      tunnel: [w1067] -> w851
      tunnel: w844 -> [w1060]
      tunnel: w843 -> [w1058]
      tunnel: w842 -> [w1056]
      tunnel: w841 -> [w1054]
      tunnel: [w1062] -> w839
      tunnel: [w1061] -> w838
      tunnel: w828 -> [w1051]
      tunnel: [w1051] -> w826
      tunnel: w825 -> [w1042]
      tunnel: w823 -> [w1045]
      tunnel: w820 -> [w1044]
      tunnel: w817 -> [w1047]
      tunnel: w814 -> [w1046]
      tunnel: w811 -> [w1038]
      tunnel: [w1047] -> w808
      tunnel: [w1046] -> w807
      tunnel: [w1045] -> w806
      tunnel: [w1044] -> w805
      tunnel: [w1043] -> w804
      tunnel: [w1042] -> w803
      tunnel: [w1041] -> w800
      tunnel: w799 -> [w1041]
      tunnel: [w1040] -> w798
      tunnel: w797 -> [w1040]
      tunnel: w770 -> [w1039]
      tunnel: [w1039] -> w768
      tunnel: [w1037] -> w756
      tunnel: w755 -> [w1037]
      frame #0 {
        n301 = Wait (ms)(milliseconds to wait=w1032) -> ()  [unwired: 1 out]
      }
      frame #1 {
        w1052 = "POS?\n"
        w1063 = u32 128 ("byte count")
        n302 = VISA Write(VISA resource name=w1060, write buffer=w1052, error in (no error)=w1058) -> (VISA resource name out=w1059:refnum<visa-resource-name>, error out=w1057:errorcluster)  [unwired: 1 out]
        n303 = VISA Write(VISA resource name=w1056, write buffer=w1052, error in (no error)=w1054) -> (VISA resource name out=w1055:refnum<visa-resource-name>, error out=w1053:errorcluster)  [unwired: 1 out]
        n304 = Number To Fractional String(number=w1038) -> (F-format string=w1050:string)  [unwired: 3 in]
        n305 = VISA Read(VISA resource name=w1059, byte count=w1063, error in (no error)=w1057) -> (VISA resource name out=w1067:refnum<visa-resource-name>, read buffer=w1062:string, error out=w1066:errorcluster)  [unwired: 1 out]
        n306 = VISA Read(VISA resource name=w1055, byte count=w1063, error in (no error)=w1053) -> (VISA resource name out=w1065:refnum<visa-resource-name>, read buffer=w1061:string, error out=w1064:errorcluster)  [unwired: 1 out]
        n307 = Concatenate Strings("MVR 1 ", w1050, "\n" ("string")) -> (w1043:string)
      }
    }
    n308 = Fract/Exp String To Number(string=w839, offset=2) -> (number=w790:dbl)  [unwired: 2 in, 1 out]
    n309 = Build Array (concatenate)(w855, w790) -> (w837:dbl[])
    n310 = Fract/Exp String To Number(string=w838, offset=2) -> (number=w789:dbl)  [unwired: 2 in, 1 out]
    n311 = Build Array (concatenate)(w836, w789) -> (w835:dbl[])
    n312 = flat-sequence {
      tunnel: w851 -> [w885]
      tunnel: w850 -> [w883]
      tunnel: [w875] -> w848
      tunnel: w849 -> [w879]
      tunnel: [w874] -> w847
      tunnel: w846 -> [w877]
      tunnel: w826 -> [w909]
      tunnel: w808 -> [w908]
      tunnel: w807 -> [w907]
      tunnel: w806 -> [w906]
      tunnel: w805 -> [w905]
      tunnel: w804 -> [w904]
      tunnel: w803 -> [w903]
      tunnel: w800 -> [w902]
      tunnel: w798 -> [w901]
      tunnel: [w894] -> w795
      tunnel: [w893] -> w788
      tunnel: [w892] -> w775
      tunnel: [w891] -> w774
      tunnel: [w890] -> w773
      tunnel: [w889] -> w772
      tunnel: w768 -> [w888]
      tunnel: [w886] -> w765
      tunnel: [w881] -> w763
      tunnel: [w880] -> w764
      tunnel: w756 -> [w873]
      frame #0 {
        n313 = flat-sequence {
          tunnel: w909 -> [w936]
          tunnel: w908 -> [w935]
          tunnel: w907 -> [w934]
          tunnel: w906 -> [w933]
          tunnel: w905 -> [w932]
          tunnel: w904 -> [w931]
          tunnel: w903 -> [w930]
          tunnel: w902 -> [w929]
          tunnel: w901 -> [w928]
          tunnel: [w927] -> w900
          tunnel: [w926] -> w899
          tunnel: [w925] -> w898
          tunnel: [w924] -> w897
          tunnel: [w923] -> w896
          tunnel: [w922] -> w895
          tunnel: [w921] -> w893
          tunnel: w888 -> [w920]
          tunnel: [w919] -> w887
          tunnel: w885 -> [w918]
          tunnel: [w916] -> w884
          tunnel: w883 -> [w917]
          tunnel: [w915] -> w882
          tunnel: w879 -> [w914]
          tunnel: [w913] -> w878
          tunnel: w877 -> [w912]
          tunnel: [w911] -> w876
          tunnel: w873 -> [w910]
          tunnel: w900 -> [w1018]
          tunnel: w899 -> [w1017]
          tunnel: w898 -> [w1005]
          tunnel: w897 -> [w1004]
          tunnel: w896 -> [w1020]
          tunnel: [w1011] -> w890
          tunnel: [w1010] -> w889
          tunnel: w895 -> [w1006]
          tunnel: [w1006] -> w894
          tunnel: [w1005] -> w892
          tunnel: [w1004] -> w891
          tunnel: w887 -> [w1003]
          tunnel: [w1003] -> w886
          tunnel: w884 -> [w1002]
          tunnel: [w1002] -> w880
          tunnel: w882 -> [w1001]
          tunnel: [w1001] -> w881
          tunnel: w878 -> [w1000]
          tunnel: w876 -> [w999]
          tunnel: [w1000] -> w875
          tunnel: [w999] -> w874
          frame #0 {
            n314 = for {
              N: w936 -> [_]
              tunnel: w935 -> [w981]
              tunnel: w934 -> [w980]
              tunnel: w933 -> [w972]
              tunnel: w932 -> [w971]
              tunnel: w931 -> [w973]
              tunnel: w930 -> [w949]
              tunnel: w929 -> [w962]
              tunnel: [w958] -> w927
              tunnel: [w957] -> w926
              tunnel: [w956] -> w925
              tunnel: [w955] -> w924
              tunnel: [w954] -> w923
              shift-right: [w953] -> w922
              shift-left: w928 -> [w959]
              tunnel: [w951] -> w921
              tunnel: w920 -> [w948]
              tunnel: [w942] -> w919
              tunnel: w918 -> [w941]
              tunnel: w917 -> [w940]
              tunnel: [w941] -> w916
              tunnel: [w940] -> w915
              tunnel: [w939] -> w913
              tunnel: w914 -> [w939]
              tunnel: w912 -> [w938]
              tunnel: [w938] -> w911
              tunnel: w910 -> [w937]
              stop <- w942 stop-if-true
              n315 = VISA Write(VISA resource name=w972, write buffer=":DATA:FRES?\n", error in (no error)=w971) -> (VISA resource name out=w969:refnum<visa-resource-name>, error out=w968:errorcluster)  [unwired: 1 out]
              n316 = VISA Write(VISA resource name=w981, write buffer="POS?\n", error in (no error)=w980) -> (VISA resource name out=w977:refnum<visa-resource-name>, error out=w976:errorcluster)  [unwired: 1 out]
              n317 = VISA Read(VISA resource name=w969, byte count=u32 128, error in (no error)=w968) -> (VISA resource name out=w964:refnum<visa-resource-name>, read buffer=w966:string, error out=w963:errorcluster)  [unwired: 1 out]
              n318 = VISA Read(VISA resource name=w977, byte count=u32 128, error in (no error)=w976) -> (VISA resource name out=w975:refnum<visa-resource-name>, read buffer=w961:string, error out=w974:errorcluster)  [unwired: 1 out]
              n319 = Fract/Exp String To Number(string=w966, offset=1) -> (number=w950:dbl)  [unwired: 2 in, 1 out]
              "Present I / A" <- w950
              n320 = Fract/Exp String To Number(string=w961, offset=2) -> (number=w954:dbl)  [unwired: 2 in, 1 out]
              n321 = Subtract(x=w937, y=w954) -> (x-y=w951:dbl)
              "Height / mm" <- w951
              n322 = Divide(x=w950, y=w962) -> (x/y=→"Present I Percent" →"Current ratio":dbl)
              n323 = Greater?(x=w950, y=w948) -> (0:w945:bool)
              n324 = Less?(x=w950, y=w949) -> (x < y?=w946:bool)
              n325 = Or(x=w946, y=w945) -> (x .or. y?=w947:bool)
              n326 = case shown="True" w947 {
                tunnel: w975 -> [w989 w994]
                tunnel: w974 -> [w988 w993]
                tunnel: w973 -> [w990 _]
                tunnel: [FALSE TRUE] -> w944
                tunnel: w964 -> [w983 w992]
                tunnel: w963 -> [w982 w991]
                tunnel: [w986 w994] -> w958
                tunnel: [w985 w993] -> w957
                tunnel: w959 -> [w984 w997]
                tunnel: w951 -> [_ w996]
                tunnel: [w984 w995] -> w953
                tunnel: [w983 w992] -> w956
                tunnel: [w982 w991] -> w955
                frame False {
                  n327 = VISA Write(VISA resource name=w989, write buffer=w990, error in (no error)=w988) -> (VISA resource name out=w986:refnum<visa-resource-name>, error out=w985:errorcluster)  [unwired: 1 out]
                }
                frame True {
                  n328 = Build Array (concatenate)(w997, w996) -> (w995:dbl[])
                }
              }
              n329 = Or(x=w944, y="stop") -> (x .or. y?=w942:bool)
            }
          }
          frame #1 {
            n330 = local read "Zvel (mm/s)"() -> (w1019:dbl)
            n331 = Divide(x=w1020, y=w1019) -> (x/y=w1007:dbl)
            n332 = Number To Fractional String(number=0) -> (F-format string=w1014:string)  [unwired: 3 in]
            n333 = Add(x=w1007, y=50) -> (x+y=w1009:dbl)
            n334 = Concatenate Strings("MOV 1 " ("string"), w1014, "\n" ("string")) -> (w1015:string)
            n335 = Wait (ms)(milliseconds to wait=w1009) -> ()  [unwired: 1 out]
            n336 = VISA Write(VISA resource name=w1018, write buffer=w1015, error in (no error)=w1017) -> (VISA resource name out=w1011:refnum<visa-resource-name>, error out=w1010:errorcluster)  [unwired: 1 out]
          }
        }
      }
    }
    n337 = Bundle(w837, w835) -> (→"Rod Pos?":cluster{dbl[], dbl[]})  [unwired: 1 in]
    n338 = Number To Fractional String(number=w788, precision (6)=i16 12) -> (F-format string=w782:string)  [unwired: 2 in]
    n339 = Number To Fractional String(number=w790, precision (6)=i16 12) -> (F-format string=w787:string)  [unwired: 2 in]
    n340 = Number To Fractional String(number=w789, precision (6)=i16 12) -> (F-format string=w784:string)  [unwired: 2 in]
    n341 = Concatenate Strings("X: ", w787, "  Y: ", w784, "  Z: ", w782, "\n" ("string")) -> (w780:string)
    n342 = Or(x=w766, y=w765) -> (x .or. y?=w767:bool)
    n343 = Write to Text File(file (use dialog)=w779, text=w780, error in=w778) -> (refnum out=w777:refnum<file>, error out=w776:errorcluster)  [unwired: 1 in, 1 out]
  }
  n344 = Close File(refnum=w16, error in=w15) -> ()  [unwired: 2 out]
  n345 = VISA Write(VISA resource name=w9, write buffer=":OUTP 0\n:SYST:ZCH ON\n", error in (no error)=w8) -> (VISA resource name out=w7:refnum<visa-resource-name>, error out=w6:errorcluster)  [unwired: 1 out]
  n346 = VISA Write(VISA resource name=w14, write buffer="ERR?\nMOV 1 0\n", error in (no error)=w13) -> (VISA resource name out=w12:refnum<visa-resource-name>, error out=w11:errorcluster)  [unwired: 1 out]
  n347 = VISA Close(VISA resource name=w7, error in (no error)=w6) -> ()  [unwired: 1 out]
  n348 = VISA Close(VISA resource name=w12, error in (no error)=w11) -> ()  [unwired: 1 out]
  n349 = flat-sequence {
    tunnel: [w1109] -> w51
    tunnel: w50 -> [w1109]
    tunnel: [w1108] -> w49
    tunnel: w48 -> [w1108]
    tunnel: [w1107] -> w47
    tunnel: w46 -> [w1107]
    tunnel: [w1106] -> w45
    tunnel: w44 -> [w1106]
    tunnel: w43 -> [w1104]
    tunnel: [w1103] -> _
    frame #0 {
      n350 = Get Date/Time In Seconds() -> (seconds since 1Jan1904=w1105:timestamp)
      n351 = Subtract(x=w1105, y=w1104) -> (x-y=w1103:dbl)
    }
  }
  n352 = Build Array(w28, w27) -> (w26:T2)
  n353 = VISA Write(VISA resource name=w47, write buffer=w59, error in (no error)=w45) -> (VISA resource name out=w56:refnum<visa-resource-name>, error out=w55:errorcluster)  [unwired: 1 out]
  n354 = VISA Write(VISA resource name=w51, write buffer=w59, error in (no error)=w49) -> (VISA resource name out=w57:refnum<visa-resource-name>, error out=w58:errorcluster)  [unwired: 1 out]
  n355 = VISA Close(VISA resource name=w56, error in (no error)=w55) -> ()  [unwired: 1 out]
  n356 = VISA Close(VISA resource name=w57, error in (no error)=w58) -> ()  [unwired: 1 out]
  n357 = call-poly <vilib>:"Plot Helper.vi"("z matrix"=w26, "y vector"=w25) -> ("3D Plot lvclass Array out"=→"Surface Scanned":refnum<class "3D Plot Datatype.lvclass">[])  [unwired: 1 in, 8 out]
